vi "Split String at Symbol.vi"(8 "error in (no error)":errorcluster, 10 "String In":string) -> (0 "error out":errorcluster, 2 "String Array Out":string[](array[string]))   [LabVIEW 2015, in "Case Manipulation.lvlib"]
uses:
  Case Manipulation.lvlib
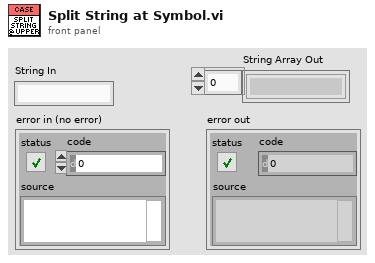
[diagram p1: front panel]
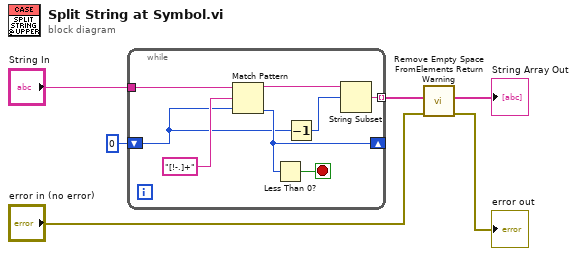
[diagram p0: block diagram]
diagram:
  n1 = while {
    tunnel: "String In" -> [w13]
    shift-right: [w11] -> _
    shift-left: 0 ("offset past match") -> [w10]
    tunnel: [w7] -> w4 mode=indexing
    stop <- w12 stop-if-true
    n2 = Match Pattern(string=w13, regular expression="[!-.]+", offset (0)=w10) -> (before substring=w9:string, offset past match=w11:i32)  [unwired: 2 out]
    n3 = Less Than 0?(x=w11) -> (x < 0?=w12:bool)
    n4 = Decrement(x=w10) -> (x-1=w8:i32)
    n5 = String Subset(string=w9, offset (0)=w8) -> (substring=w7:string)  [unwired: 1 in]
  }
  n6 = call "Remove Empty Space FromElements Return Warning.vi"("error in (no error)"="error in (no error)", "String Array In"=w4) -> ("error out"=→"error out":errorcluster, "String Array Out"=→"String Array Out":string[])  [unwired: 8 in]
